vi "Add Minor Frame.vi"(7 "minorFramePeriod":i32, 8 "error in":errorcluster, 9 "messageRefs":string[](array[string]), 10 "name":string, 11 "channel in":refnum<k24>) -> (0 "error out":errorcluster, 2 "new minor frame":refnum<k24>, 3 "channel out":refnum<k24>)   [LabVIEW 2020, in "Ballard_1553_Parameter_ni.lvlib"]
uses:
  Ballard_1553_Parameter_ni.lvlib
  C:/Users/Administrator/Desktop/GIT/Ballard-Arinc-429-XML-Generator/Source/Assemblies/Aim_1553_Parameter_ni/bin/Debug/AIM_1553_Parameter_ni.dll
  Assemblies/Aim_1553_Parameter_ni/bin/Debug/AIM_1553_Parameter_ni.dll
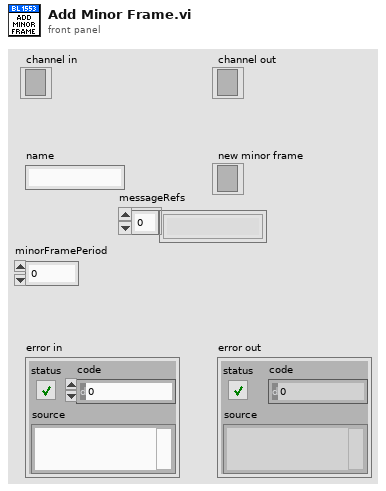
[diagram p1: front panel]
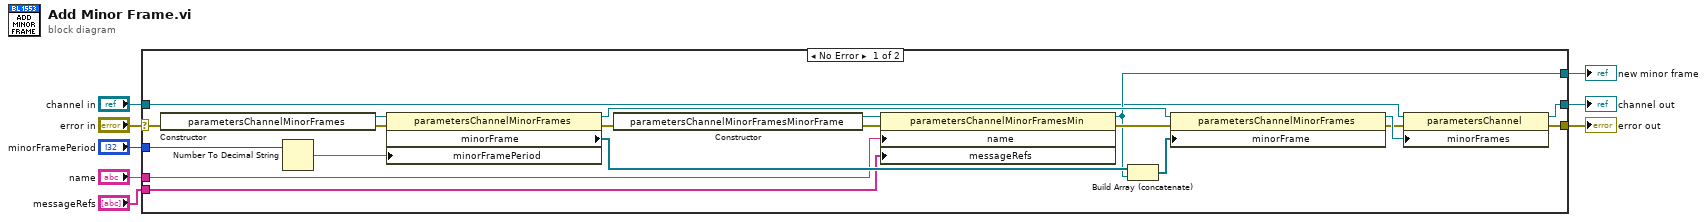
[diagram p0: block diagram]
diagram:
  n1 = case shown="No Error" "error in" {
    selector: "error in" -> [w12 w29]
    tunnel: [w28 w30] -> w8
    tunnel: [w27 w29] -> w7
    tunnel: "channel in" -> [w9 w30]
    tunnel: [w17 _] -> w4
    tunnel: "name" -> [w16 _]
    tunnel: "minorFramePeriod" -> [w15 _]
    tunnel: "messageRefs" -> [w13 _]
    frame No Error {
      n2 = constructor class="parametersChannelMinorFrames"(error in=w12) -> (reference out=w10:refnum<k24>, error out=w11:errorcluster)  [unwired: 2 in, 1 out]
      n3 = Number To Decimal String(number=w15) -> (decimal integer string=w14:string)  [unwired: 1 in]
      n4 = property class="parametersChannelMinorFrames"(reference=w10, error in=w11, "minorFramePeriod"=w14) -> (reference out=w23:refnum<k24>, error out=w21:errorcluster, "minorFrame"=w24:refnum<k24>[])
      n5 = constructor class="parametersChannelMinorFramesMin"(error in=w21) -> (reference out=w25:refnum<k24>, error out=w26:errorcluster)  [unwired: 2 in, 1 out]
      n6 = property class="parametersChannelMinorFramesMin"(reference=w25, error in=w26, "name"=w16, "messageRefs"=w13) -> (reference out=w17:refnum<k24>, error out=w20:errorcluster)
      n7 = Build Array (concatenate)(w24, w17) -> (w22:refnum<k24>[])
      n8 = property class="parametersChannelMinorFrames"(reference=w23, error in=w20, "minorFrame"=w22) -> (reference out=w19:refnum<k24>, error out=w18:errorcluster)
      n9 = property class="parametersChannel"(reference=w9, error in=w18, "minorFrames"=w19) -> (reference out=w28:refnum<k24>, error out=w27:errorcluster)
    }
    frame Error {
    }
  }
  "channel out" <- w8
  "error out" <- w7
  "new minor frame" <- w4
